vi "ReadDataMethod.vi"(8 "Error In":errorcluster, 11 "object in":refnum<class "DataType.lvclass">) -> (0 "Error Out":errorcluster, 2 "Data Method":refnum<class "IDataMethod.lvclass">, 3 "object out":refnum<class "DataType.lvclass">)   [LabVIEW 2024, in "DataType.lvclass"]
uses:
  DataType.lvclass
  IDataMethod_interface/IDataMethod.lvclass
  DataType.lvclass/DataType.ctl
panel:
  # "Connector Pane"
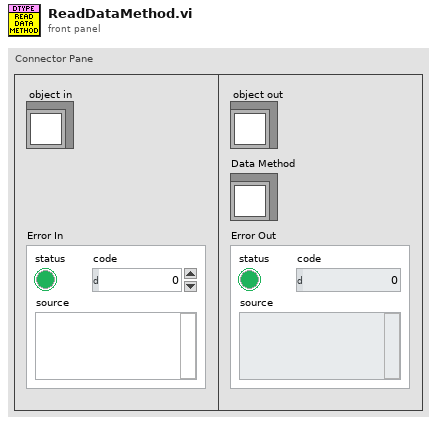
[diagram p1: front panel]
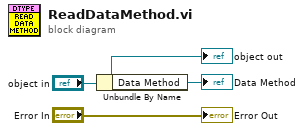
[diagram p0: block diagram]
diagram:
  n1 = Unbundle By Name("object in") -> ("Data Method"=→"Data Method":refnum<class "IDataMethod.lvclass">)
  "Error Out" <- "Error In"
  "object out" <- "object in"
